vi "Program1.vi"   [LabVIEW 2016, in "Program1.lvrbt"]
uses:
  Program1.lvrbt
  <vilib>/NXT/LegoClasses/BrickReference/BrickReference.lvclass
  <vilib>/NXT/Subs/LVHSConnector.ctl
  <vilib>/NXT/NXTIO Xnodes/NXTIOXNode/NXTIO.xnode
  <vilib>/NXT/NXTIO Xnodes/AddressXNode/NXTIOAddress.xnode
  <vilib>/NXT/Hardware/Plugins/Tetrix DC Motor/TetrixDCMotorAddress.ctl
  <vilib>/NXT/NXTIO Xnodes/NXTIONodeSubVIs/TETRIX IO Move DC Motors.vi
  <vilib>/NXT/Dual Mode Library/Waits/Wait_Num.vi
  <vilib>/NXT/Subs/ColorSensorColors.ctl
  <vilib>/NXT/Block Support/NXT_InputPort.ctl
  <vilib>/NXT/Dual Mode Library/Sensors/EV3_Color_Color.vi
  <vilib>/NXT/Hardware/Plugins/Tetrix 180 deg Servo/Tetrix180ServoAddress.ctl
  <vilib>/NXT/NXTIO Xnodes/NXTIONodeSubVIs/TETRIX IO Move Servos.vi
types:
  T1 = typedef "TetrixDCMotorAddress.ctl" = i32
  T2 = typedef "LVHSConnector.ctl" = refnum<class "BrickReference.lvclass">
  T3 = cluster{"TetrixDCMotor":T1, "TetrixDCMotor 2":T1}
  T4 = typedef "NXT_InputPort.ctl" = u32
  T5 = typedef "ColorSensorColors.ctl" = enum16{"No Color", "Black", "Blue", "Green", "Yellow", "Red", "White", "Brown"}
  T6 = typedef "Tetrix180ServoAddress.ctl" = i32
  T7 = cluster{"Tetrix180Servo":T6, "Tetrix180Servo":T6}
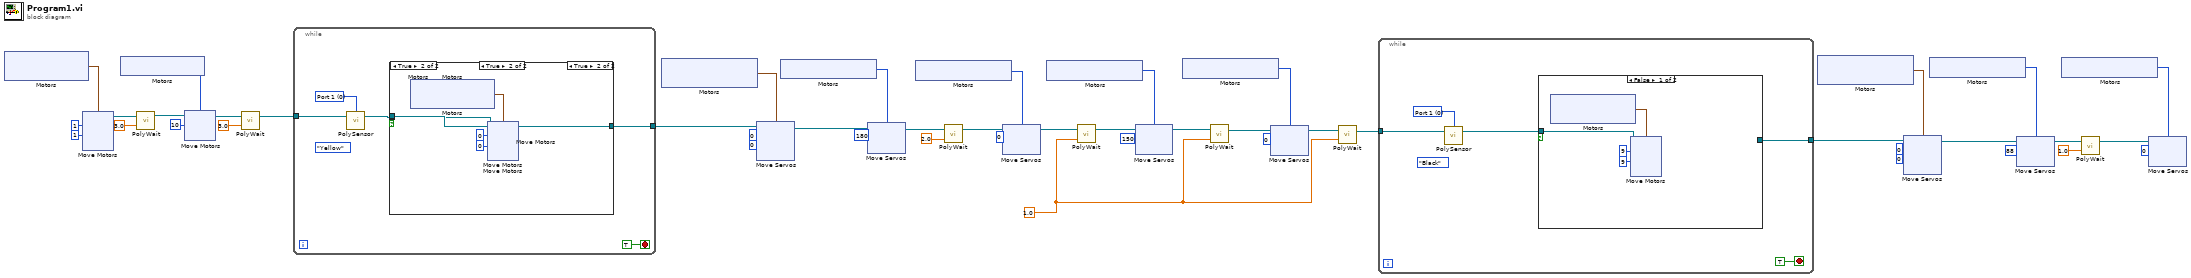
[diagram p0: block diagram]
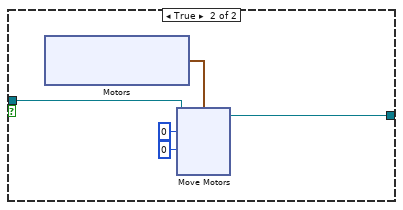
[diagram p2: hidden frame]
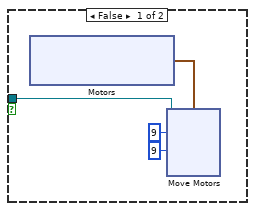
[diagram p3: hidden frame]
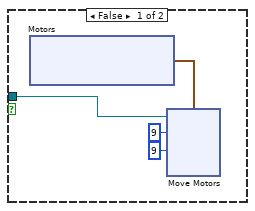
[diagram p4: hidden frame]
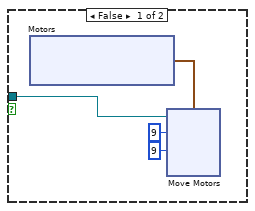
[diagram p5: hidden frame]
diagram:
  w15 = sgl 1.0 ("Time (1 sec)")
  n1 = xnode "Motors"() -> ("Motor"=w46:cluster{"TetrixDCMotor":T1, "TetrixDCMotor":T1})
  n2 = xnode "Move Motors"("Power/Speed 2"=i8 1, "Power/Speed 1"=i8 1, "Motors"=w46) -> ("NXT/EV3"=w43:T2)  [unwired: 1 in]
  n3 = xnode "Motors"() -> ("Motor"=w39:T1)
  n4 = call-poly <vilib>:"PolyWait.vi"("Time (1 sec)"=sgl 3.0, "NXT/EV3"=w43) -> ("NXT/EV3"=w41:T2)  [unwired: 2 in]
  n5 = xnode "Move Motors"("Power/Speed 1"=i8 10, "Motors"=w39, "NXT/EV3"=w41) -> ("NXT/EV3"=w38:T2)
  n6 = call-poly <vilib>:"PolyWait.vi"("Time (1 sec)"=sgl 3.0, "NXT/EV3"=w38) -> ("NXT/EV3"=w36:T2)  [unwired: 2 in]
  n7 = while {
    tunnel: w36 -> [w51]
    tunnel: [w48] -> w35
    stop <- TRUE stop-if-true
    w50 = T4 0 items=["Port 1", "Port 2", "Port 3", "Port 4"] ("Port (Port 1)")
    (unwired) ColorSensorColors."Yellow" ("Detected Color")
    n8 = call-poly <vilib>:"PolySensor.vi"("NXT/EV3"=w51, "Port (Port 1)"=w50) -> ("NXT/EV3"=w47:T2)  [unwired: 1 in, 1 out]
    n9 = case shown="True" {
      selector: _ -> [_ _]
      tunnel: [_ w66] -> _
      tunnel: w47 -> [w52 w65]
      frame False {
        n10 = xnode "Motors"() -> ("Motor"=w55:cluster{"TetrixDCMotor":T1, "TetrixDCMotor":T1})
        n11 = xnode "Move Motors"("Power/Speed 2"=i8 9, "Power/Speed 1"=i8 9, "Motors"=w55, "NXT/EV3"=w52) -> ()  [unwired: 1 out]
      }
      frame True {
        n12 = xnode "Motors"() -> ("Motor"=w69:cluster{"TetrixDCMotor":T1, "TetrixDCMotor":T1})
        n13 = xnode "Move Motors"("Power/Speed 2"=i8 0, "Power/Speed 1"=i8 0, "Motors"=w69, "NXT/EV3"=w65) -> ("NXT/EV3"=w66:T2)
      }
    }
    n14 = case shown="True" {
      selector: _ -> [_ _]
      tunnel: _ -> [w81 w92]
      tunnel: [_ w93] -> _
      frame False {
        n15 = xnode "Motors"() -> ("Motor"=w82:cluster{"TetrixDCMotor":T1, "TetrixDCMotor":T1})
        n16 = xnode "Move Motors"("Power/Speed 2"=i8 9, "Power/Speed 1"=i8 9, "Motors"=w82, "NXT/EV3"=w81) -> ()  [unwired: 1 out]
      }
      frame True {
        n17 = xnode "Motors"() -> ("Motor"=w96:cluster{"TetrixDCMotor":T1, "TetrixDCMotor":T1})
        n18 = xnode "Move Motors"("Power/Speed 2"=i8 0, "Power/Speed 1"=i8 0, "Motors"=w96, "NXT/EV3"=w92) -> ("NXT/EV3"=w93:T2)
      }
    }
    n19 = case shown="True" {
      selector: _ -> [_ _]
      tunnel: _ -> [w108 w119]
      tunnel: [_ w120] -> w48
      frame False {
        n20 = xnode "Motors"() -> ("Motor"=w109:cluster{"TetrixDCMotor":T1, "TetrixDCMotor":T1})
        n21 = xnode "Move Motors"("Power/Speed 2"=i8 9, "Power/Speed 1"=i8 9, "Motors"=w109, "NXT/EV3"=w108) -> ()  [unwired: 1 out]
      }
      frame True {
        n22 = xnode "Motors"() -> ("Motor"=w123:cluster{"TetrixDCMotor":T1, "TetrixDCMotor":T1})
        n23 = xnode "Move Motors"("Power/Speed 2"=i8 0, "Power/Speed 1"=i8 0, "Motors"=w123, "NXT/EV3"=w119) -> ("NXT/EV3"=w120:T2)
      }
    }
  }
  n24 = xnode "Motors"() -> ("Motor"=w33:T7)
  n25 = xnode "Move Servos"("Position 2"=u8 0, "Position 1"=u8 0, "Motors"=w33, "NXT/EV3"=w35) -> ("NXT/EV3"=w31:T2)
  n26 = xnode "Motors"() -> ("Motor"=w29:T6)
  n27 = xnode "Move Servos"("Position 1"=u8 180, "Motors"=w29, "NXT/EV3"=w31) -> ("NXT/EV3"=w28:T2)
  n28 = xnode "Motors"() -> ("Motor"=w26:T6)
  n29 = call-poly <vilib>:"PolyWait.vi"("Time (1 sec)"=sgl 2.0, "NXT/EV3"=w28) -> ("NXT/EV3"=w24:T2)  [unwired: 2 in]
  n30 = xnode "Move Servos"("Position 1"=u8 0, "Motors"=w26, "NXT/EV3"=w24) -> ("NXT/EV3"=w23:T2)
  n31 = xnode "Motors"() -> ("Motor"=w20:T6)
  n32 = call-poly <vilib>:"PolyWait.vi"("Time (1 sec)"=w15, "NXT/EV3"=w23) -> ("NXT/EV3"=w22:T2)  [unwired: 2 in]
  n33 = xnode "Move Servos"("Position 1"=u8 150, "Motors"=w20, "NXT/EV3"=w22) -> ("NXT/EV3"=w19:T2)
  n34 = xnode "Motors"() -> ("Motor"=w18:T6)
  n35 = call-poly <vilib>:"PolyWait.vi"("Time (1 sec)"=w15, "NXT/EV3"=w19) -> ("NXT/EV3"=w16:T2)  [unwired: 2 in]
  n36 = xnode "Move Servos"("Position 1"=u8 0, "Motors"=w18, "NXT/EV3"=w16) -> ("NXT/EV3"=w14:T2)
  n37 = call-poly <vilib>:"PolyWait.vi"("Time (1 sec)"=w15, "NXT/EV3"=w14) -> ("NXT/EV3"=w13:T2)  [unwired: 2 in]
  n38 = while {
    tunnel: w13 -> [w135]
    tunnel: [w136] -> w12
    stop <- TRUE stop-if-true
    w133 = T4 0 items=["Port 1", "Port 2", "Port 3", "Port 4"] ("Port (Port 1)")
    (unwired) ColorSensorColors."Black" ("Detected Color")
    n39 = call-poly <vilib>:"PolySensor.vi"("NXT/EV3"=w135, "Port (Port 1)"=w133) -> ("NXT/EV3"=w134:T2)  [unwired: 1 in, 1 out]
    n40 = case shown="False" {
      selector: _ -> [_ _]
      tunnel: [_ w152] -> w136
      tunnel: w134 -> [w138 w151]
      frame False {
        n41 = xnode "Motors"() -> ("Motor"=w141:cluster{"TetrixDCMotor":T1, "TetrixDCMotor":T1})
        n42 = xnode "Move Motors"("Power/Speed 2"=i8 9, "Power/Speed 1"=i8 9, "Motors"=w141, "NXT/EV3"=w138) -> ()  [unwired: 1 out]
      }
      frame True {
        n43 = xnode "Motors"() -> ("Motor"=w155:cluster{"TetrixDCMotor":T1, "TetrixDCMotor":T1})
        n44 = xnode "Move Motors"("Power/Speed 2"=i8 0, "Power/Speed 1"=i8 0, "Motors"=w155, "NXT/EV3"=w151) -> ("NXT/EV3"=w152:T2)
      }
    }
  }
  n45 = xnode "Motors"() -> ("Motor"=w10:T7)
  n46 = xnode "Move Servos"("Position 2"=u8 0, "Position 1"=u8 0, "Motors"=w10, "NXT/EV3"=w12) -> ("NXT/EV3"=w8:T2)
  n47 = xnode "Motors"() -> ("Motor"=w6:T6)
  n48 = xnode "Move Servos"("Position 1"=u8 88, "Motors"=w6, "NXT/EV3"=w8) -> ("NXT/EV3"=w5:T2)
  n49 = xnode "Motors"() -> ("Motor"=w3:T6)
  n50 = call-poly <vilib>:"PolyWait.vi"("Time (1 sec)"=sgl 1.0, "NXT/EV3"=w5) -> ("NXT/EV3"=w1:T2)  [unwired: 2 in]
  n51 = xnode "Move Servos"("Position 1"=u8 0, "Motors"=w3, "NXT/EV3"=w1) -> ()  [unwired: 1 out]
